vi "VI Tree.vi"   [LabVIEW 2020, in "Keithley 27XX.lvlib"]
uses:
  Keithley 27XX.lvlib
  Action-Status/Close Channel.vi
  Configure/Measurement Specific/Configure Thermocouple.vi
  Data/Read Multiple Direct.vi
panel:
  # "© 2005 National Instruments Corporation.  ALL RIGHTS RESERVED."
  # "VI TREE"
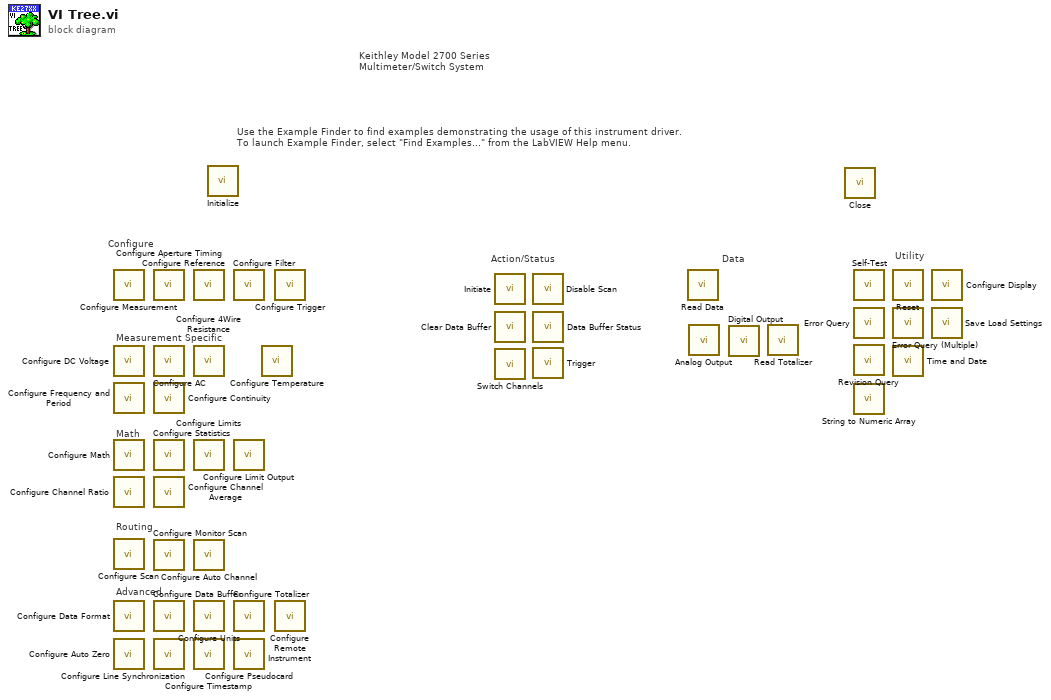
[diagram p0: block diagram]
diagram:
  # "Keithley Model 2700 Series\nMultimeter/Switch System"
  # "Configure"
  # "Advanced"
  # "Routing"
  # "Use the Example Finder to find examples demonstrating the usage of this instrument driver.\nTo launch Example Finder, select \"Find Examples...\" from the LabVIEW Help menu."
  # "Data"
  # "Math"
  # "Measurement Specific"
  # "Action/Status"
  # "Utility"
  n1 = call "Configure Measurement.vi"() -> ()  [unwired: 14 in, 2 out]
  n2 = call "Configure DC Voltage.vi"() -> ()  [unwired: 14 in, 2 out]
  n3 = call "Configure Frequency and Period.vi"() -> ()  [unwired: 14 in, 2 out]
  n4 = call "Configure Math.vi"() -> ()  [unwired: 18 in, 2 out]
  n5 = call "Configure Channel Ratio.vi"() -> ()  [unwired: 14 in, 2 out]
  n6 = call "Configure Scan.vi"() -> ()  [unwired: 14 in, 2 out]
  n7 = call "Configure Data Format.vi"() -> ()  [unwired: 14 in, 2 out]
  n8 = call "Configure Auto Zero.vi"() -> ()  [unwired: 14 in, 2 out]
  n9 = call "Configure Aperture Timing.vi"() -> ()  [unwired: 14 in, 2 out]
  n10 = call "Configure AC.vi"() -> ()  [unwired: 14 in, 2 out]
  n11 = call "Configure Continuity.vi"() -> ()  [unwired: 14 in, 2 out]
  n12 = call "Configure Statistics.vi"() -> ()  [unwired: 14 in, 2 out]
  n13 = call "Configure Channel Average.vi"() -> ()  [unwired: 14 in, 2 out]
  n14 = call "Configure Monitor Scan.vi"() -> ()  [unwired: 14 in, 2 out]
  n15 = call "Configure Data Buffer.vi"() -> ()  [unwired: 14 in, 2 out]
  n16 = call "Configure Line Synchronization.vi"() -> ()  [unwired: 14 in, 2 out]
  n17 = call "Configure Reference.vi"() -> ()  [unwired: 14 in, 2 out]
  n18 = call "Configure 4Wire Resistance.vi"() -> ()  [unwired: 14 in, 2 out]
  n19 = call "Configure Limits.vi"() -> ()  [unwired: 18 in, 2 out]
  n20 = call "Configure Auto Channel.vi"() -> ()  [unwired: 14 in, 2 out]
  n21 = call "Configure Units.vi"() -> ()  [unwired: 14 in, 2 out]
  n22 = call "Configure Timestamp.vi"() -> ()  [unwired: 14 in, 2 out]
  n23 = call "Initialize.vi"() -> ()  [unwired: 14 in, 2 out]
  n24 = call "Configure Filter.vi"() -> ()  [unwired: 14 in, 2 out]
  n25 = call "Configure Limit Output.vi"() -> ()  [unwired: 14 in, 2 out]
  n26 = call "Configure Totalizer.vi"() -> ()  [unwired: 14 in, 2 out]
  n27 = call "Configure Pseudocard.vi"() -> ()  [unwired: 14 in, 2 out]
  n28 = call-poly "Configure Temperature.vi"() -> ()  [unwired: 18 in, 2 out]
  n29 = call "Configure Trigger.vi"() -> ()  [unwired: 14 in, 2 out]
  n30 = call "Configure Remote Instrument.vi"() -> ()  [unwired: 14 in, 2 out]
  n31 = call "Initiate.vi"() -> ()  [unwired: 14 in, 2 out]
  n32 = call "Clear Data Buffer.vi"() -> ()  [unwired: 14 in, 2 out]
  n33 = call-poly "Switch Channels.vi"() -> ()  [unwired: 14 in, 2 out]
  n34 = call "Disable Scan.vi"() -> ()  [unwired: 14 in, 2 out]
  n35 = call "Data Buffer Status.vi"() -> ()  [unwired: 11 in, 5 out]
  n36 = call "Trigger.vi"() -> ()  [unwired: 14 in, 2 out]
  n37 = call-poly "Read Data.vi"() -> ()  [unwired: 10 in, 6 out]
  n38 = call "Analog Output.vi"() -> ()  [unwired: 14 in, 2 out]
  n39 = call "Digital Output.vi"() -> ()  [unwired: 14 in, 2 out]
  n40 = call "Read Totalizer.vi"() -> ()  [unwired: 13 in, 3 out]
  n41 = call "Close.vi"() -> ()  [unwired: 15 in, 1 out]
  n42 = call "Self-Test.vi"() -> ()  [unwired: 12 in, 4 out]
  n43 = call "Error Query.vi"() -> ()  [unwired: 12 in, 4 out]
  n44 = call "Revision Query.vi"() -> ()  [unwired: 8 in, 4 out]
  n45 = call "String to Numeric Array.vi"() -> ()  [unwired: 11 in, 1 out]
  n46 = call "Reset.vi"() -> ()  [unwired: 14 in, 2 out]
  n47 = call "Error Query (Multiple).vi"() -> ()  [unwired: 12 in, 4 out]
  n48 = call "Time and Date.vi"() -> ()  [unwired: 14 in, 2 out]
  n49 = call "Configure Display.vi"() -> ()  [unwired: 14 in, 2 out]
  n50 = call "Save Load Settings.vi"() -> ()  [unwired: 14 in, 2 out]
